vi "RSZVB Get Coherent Signal State.vi"(8 "error in (no error)":errorcluster {"code" format="%.0x"}, 9 "Port (1)":i32=1, 10 "Channel (1)":i32=1, 11 "VISA session":refnum<visa-resource-name>) -> (0 "error out":errorcluster {"code" format="%.0x"}, 1 "Coherent Signal":bool, 3 "dup VISA session":refnum<visa-resource-name>)   [LabVIEW 2011]
doc: "This VI returns whether the signal at port no. <Pt> is a coherent or a non-coherent signal.\n\nNote(s):\n\n(1) This VI is not available for R&S ZVB instrument.\n\nRemote-control command(s):\nSOURce<Ch>:CMODe:PORT<Pt>[:STATe]?"
uses:
  _utility/RSZVB Global Data.vi
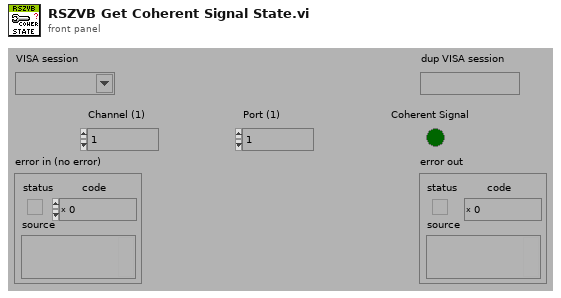
[diagram p1: front panel]
types:
  T1 = cluster{"Error Checking (T: On)":bool, "Installed Options":string[], "Data Valid?":bool, "Ports":i32, "Model":string[], "Option Checking (T: On)":bool}[]
  T2 = cluster{"Error Checking (T: On)":bool, "Installed Options":string[], "Data Valid?":bool, "Ports":i32, "Model":string[], "Option Checking (T: On)":bool}
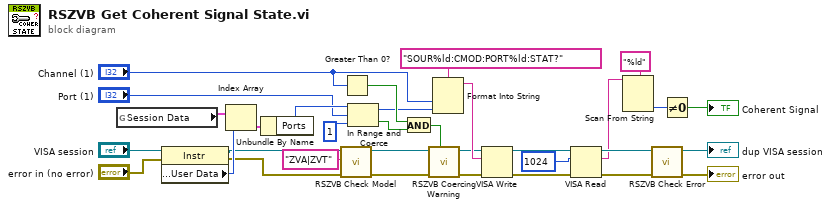
[diagram p0: block diagram]
diagram:
  n1 = global read "RSZVB Global Data.vi" "Session Data"() -> (w26:T1)
  n2 = property class="Instr"(reference="VISA session", error in="error in (no error)") -> (reference out=w2:refnum<visa-resource-name>, error out=w1:errorcluster, "General Settings:User Data"=w24:u32)
  n3 = Index Array(array=w26, index=w24) -> (element=w27:T2)
  n4 = Unbundle By Name(w27) -> ("Ports"=w23:i32)
  n5 = call "RSZVB Check Model.vi"("error in (no error)"=w1, "Model"="ZVA|ZVT", "VISA session"=w2) -> ("error out"=w3:errorcluster, "dup VISA session"=w4:refnum<visa-resource-name>)  [unwired: 7 in]
  n6 = Greater Than 0?(x="Channel (1)") -> (x > 0?=w33:bool)
  n7 = In Range and Coerce(upper limit=w23, x="Port (1)", lower limit=1) -> (coerced(x)=w22:i32, In Range?=w32:bool)
  n8 = And(x=w33, y=w32) -> (x .and. y?=w21:bool)
  n9 = call "RSZVB Coercing Warning.vi"("In Range?"=w21, "error in (no error)"=w3, "VISA session"=w4) -> ("error out"=w30:errorcluster, "dup VISA session"=w29:refnum<visa-resource-name>)  [unwired: 7 in]
  n10 = Format Into String(format string="SOUR%ld:CMOD:PORT%ld:STAT?", "Channel (1)", w22) -> (resulting string=w31:string)  [unwired: 2 in, 1 out]
  n11 = VISA Write(VISA resource name=w29, write buffer=w31, error in (no error)=w30) -> (VISA resource name out=w13:refnum<visa-resource-name>, error out=w12:errorcluster)  [unwired: 1 out]
  n12 = VISA Read(VISA resource name=w13, byte count=u32 1024 ("byte count (0)"), error in (no error)=w12) -> (VISA resource name out=w15:refnum<visa-resource-name>, read buffer=w6:string, error out=w16:errorcluster)  [unwired: 1 out]
  n13 = Scan From String(format string="%ld", input string=w6) -> (output 1=w8:i32)  [unwired: 3 in, 3 out]
  n14 = call "RSZVB Check Error.vi"("error in (no error)"=w16, "VISA session"=w15) -> ("error out"=→"error out":errorcluster, "dup VISA session"=→"dup VISA session":refnum<visa-resource-name>)  [unwired: 8 in]
  n15 = Not Equal To 0?(x=w8) -> (x != 0?=→"Coherent Signal":bool)
